vi "Euler_(SubVI).vi"(9 "XYZ":dbl[](array[numeric]) format="%0.2f", 10 "Euler angles":T2) -> (0 "POSE":dbl[](array[numeric]), 1 "RPY":cluster{"roll":dbl, "pitch":dbl, "yaw":dbl}, 2 "noa":cluster{T1, T1, T1}, 3 "Rotation matrix":dbl[][](array[numeric]))   [LabVIEW 2015]
uses:
  <vilib>/Analysis/Matrix/Datatypes/RealMatrix.ctl
  <vilib>/robotics/Kinematics/NI_Kinematics.lvlib
  <resource>/lvanlys.dll
  <vilib>/Analysis/Matrix/NI_Matrix.lvlib
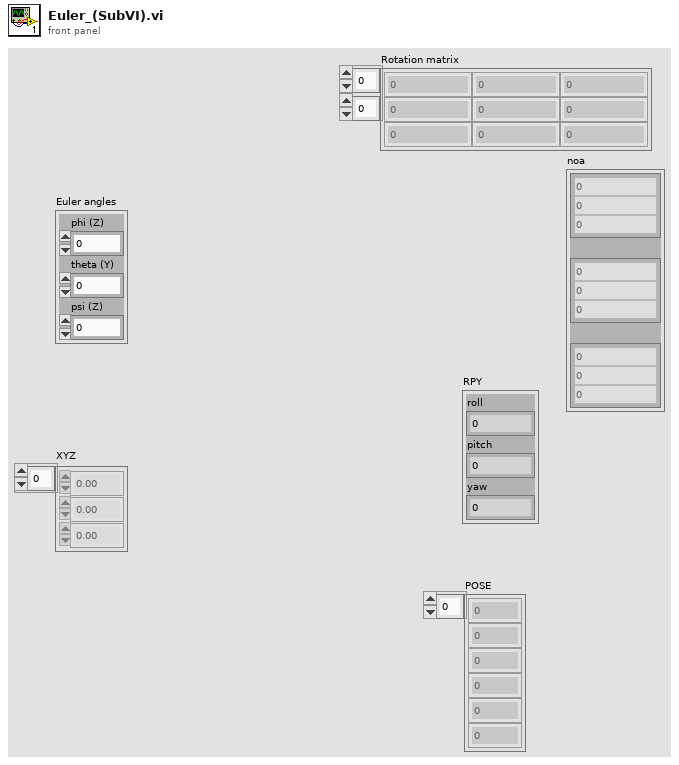
[diagram p1: front panel]
types:
  T1 = typedef "NI_Matrix.lvlib/RealMatrix.ctl" = dbl[][]
  T2 = cluster{"phi (Z)":dbl, "theta (Y)":dbl, "psi (Z)":dbl}
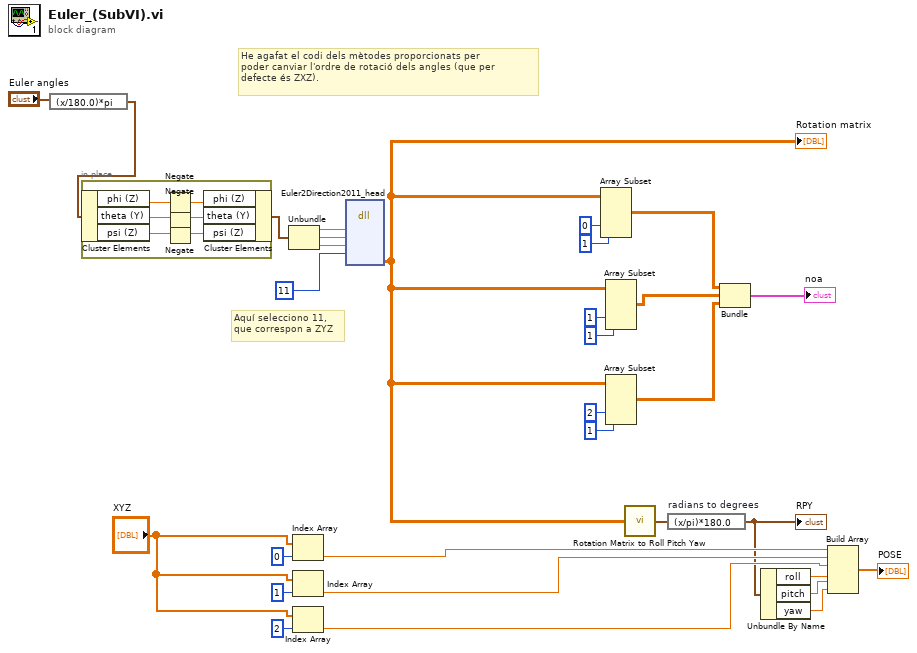
[diagram p0: block diagram]
diagram:
  # "Aquí selecciono 11,\nque correspon a ZYZ"
  # "He agafat el codi dels mètodes proporcionats per\npoder canviar l'ordre de rotació dels angles (que per\ndefecte és ZXZ)."
  n1 = expression code="(x/180.0)*pi" ("degrees to radians")("Euler angles") -> (w2:T2)
  n2 = in-place {
    n3 = in-place-cluster #1(w2) -> ("phi (Z)"=w36:dbl, "theta (Y)"=w37:dbl, "psi (Z)"=w35:dbl)
    n4 = Negate(x=w36) -> (-x=w32:dbl)
    n5 = Negate(x=w37) -> (-x=w33:dbl)
    n6 = Negate(x=w35) -> (-x=w34:dbl)
    n7 = in-place-cluster #1("phi (Z)"=w32, "theta (Y)"=w33, "psi (Z)"=w34) -> (w3:T2)
  }
  n8 = Unbundle(w3) -> ("phi (Z)"=w7:dbl, "theta (Y)"=w6:dbl, "psi (Z)"=w5:dbl)
  n9 = Index Array(array="XYZ", index=0) -> (element=w27:dbl)
  n10 = Index Array(array="XYZ", index=1) -> (element=w26:dbl)
  n11 = Index Array(array="XYZ", index=2) -> (element=w25:dbl)
  n12 = dll-call lib="C:/Program Files (x86)/National Instruments/LabVIEW 2015/resource/lvanlys.*" fn="Euler2Direction2011_head"("phi"=w7, "theta"=w6, "psi"=w5, "rotateOrder"=11) -> ("direction"=w4:dbl[][])  [unwired: 9 in, 2 out]
  "Rotation matrix" <- w4
  n13 = Array Subset(array=w4, index (col)=0 ("index"), length (col)=1 ("length")) -> (w11:dbl[][])  [unwired: 2 in]
  n14 = Array Subset(array=w4, index (col)=1 ("index"), length (col)=1 ("length")) -> (w10:dbl[][])  [unwired: 2 in]
  n15 = Array Subset(array=w4, index (col)=2 ("index"), length (col)=1 ("length")) -> (w9:dbl[][])  [unwired: 2 in]
  n16 = call <vilib>:"Rotation Matrix to Roll Pitch Yaw.vi"("rotation matrix"=w4) -> ("angles"=w31:cluster{"roll":dbl, "pitch":dbl, "yaw":dbl})
  n17 = expression code="(x/pi)*180.0" "radians to degrees"(w31) -> (w19:cluster{"roll":dbl, "pitch":dbl, "yaw":dbl})
  "RPY" <- w19
  n18 = Bundle(w11, w10, w9) -> (→"noa":cluster{dbl[][], dbl[][], dbl[][]})  [unwired: 1 in]
  n19 = Unbundle By Name(w19) -> ("roll"=w28:dbl, "pitch"=w29:dbl, "yaw"=w30:dbl)
  n20 = Build Array(w27, w26, w25, w28, w29, w30) -> (→"POSE":dbl[])
